vi "Load And Parse Bitfile Test.vi"() -> ()   [LabVIEW 2018]
uses:
  <vilib>/rvi/DataTransferAndStorage/Container/XNode/niFpgaContainer.xnode
  <vilib>/rvi/interface/RandomDataEmulation/nirviRandomDataFpgaReadWriteTemplate.vi
panel:
  out "Fast timeout 3":bool
  out "Fast timeout 2":bool
  in  "Group1.I16":i16
  in  "Group1.I8":i8
  in  "Group1.I64":i64
  in  "Group1.I32":i32
  in  "Group1.U16":u16
  in  "Group1.U8":u8
  in  "Group1.U64":u64
  in  "Group1.U32":u32
  in  "Group1.SGL":sgl
  in  "Group2.Boolean":bool
  out "Group1.I16 out":i16
  out "Group1.I8 out":i8
  out "Group1.I64 out":i64
  out "Group1.I32 out":i32
  out "Group1.U16 out":u16
  out "Group1.U8 out":u8
  out "Group1.U64 out":u64
  out "Group1.U32 out":u32
  out "Group1.SGL out":sgl
  out "Group2.Boolean out":bool
  in  "Group2.FXP24.5":fxp<+/-,24,5>
  in  "Group2.FXP16.5":fxp<+/-,16,5>
  in  "Group2.FXP32.8":fxp<+/-,32,8>
  in  "Group2.FXP64.32":fxp<+/-,64,32>
  out "Group2.FXP24.5 out":fxp<+/-,24,5>
  out "Group2.FXP16.5 out":fxp<+/-,16,5>
  out "Group2.FXP32.8 out":fxp<+/-,32,8>
  out "Group2.FXP64.32 out":fxp<+/-,64,32>
  in  "Group2.FXP16.7":fxp<+/-,16,7>
  out "Group2.FXP16.7 out":fxp<+/-,16,7>
  in  "Group2.FXP20.5":fxp<+/-,20,5>
  out "Group2.FXP20.5 out":fxp<+/-,20,5>
  in  "Group2.FXP27.5":fxp<+/-,27,5>
  out "Group2.FXP27.5 out":fxp<+/-,27,5>
  in  "Group2.FXP32.16":fxp<+/-,32,16>
  out "Group2.FXP32.16 out":fxp<+/-,32,16>
  in  "Group2.FXP16.3":fxp<+,16,3>
  out "Group2.FXP16.3 out":fxp<+,16,3>
  in  "Group2.FXP18.3":fxp<+,18,3>
  out "Group2.FXP18.3 out":fxp<+,18,3>
  in  "FXP18.3":fxp<+,18,3>
  out "FXP18.3 out":fxp<+,18,3>
  in  "FXP16.3":fxp<+,16,3>
  out "FXP16.3 out":fxp<+,16,3>
  in  "FXP32.16":fxp<+/-,32,16>
  out "FXP32.16 out":fxp<+/-,32,16>
  in  "FXP27.5":fxp<+/-,27,5>
  out "FXP27.5 out":fxp<+/-,27,5>
  in  "FXP20.5":fxp<+/-,20,5>
  out "FXP20.5 out":fxp<+/-,20,5>
  in  "FXP16.7":fxp<+/-,16,7>
  out "FXP16.7 out":fxp<+/-,16,7>
  out "FXP64.32 out":fxp<+/-,64,32>
  out "FXP32.8 out":fxp<+/-,32,8>
  out "FXP16.5 out":fxp<+/-,16,5>
  out "FXP24.5 out":fxp<+/-,24,5>
  in  "FXP64.32":fxp<+/-,64,32>
  in  "FXP32.8":fxp<+/-,32,8>
  in  "FXP16.5":fxp<+/-,16,5>
  in  "FXP24.5":fxp<+/-,24,5>
  out "Fast timeout":bool
  out "Med timeout":bool
  out "Slow timeout":bool
  in  "I16":i16
  in  "I8":i8
  in  "I64":i64
  in  "I32":i32
  in  "U16":u16
  in  "U8":u8
  in  "U64":u64
  in  "U32":u32
  in  "SGL":sgl
  in  "Boolean":bool
  out "I16 out":i16
  out "I8 out":i8
  out "I64 out":i64
  out "I32 out":i32
  out "U16 out":u16
  out "U8 out":u8
  out "U64 out":u64
  out "U32 out":u32
  out "SGL out":sgl
  out "Boolean out":bool
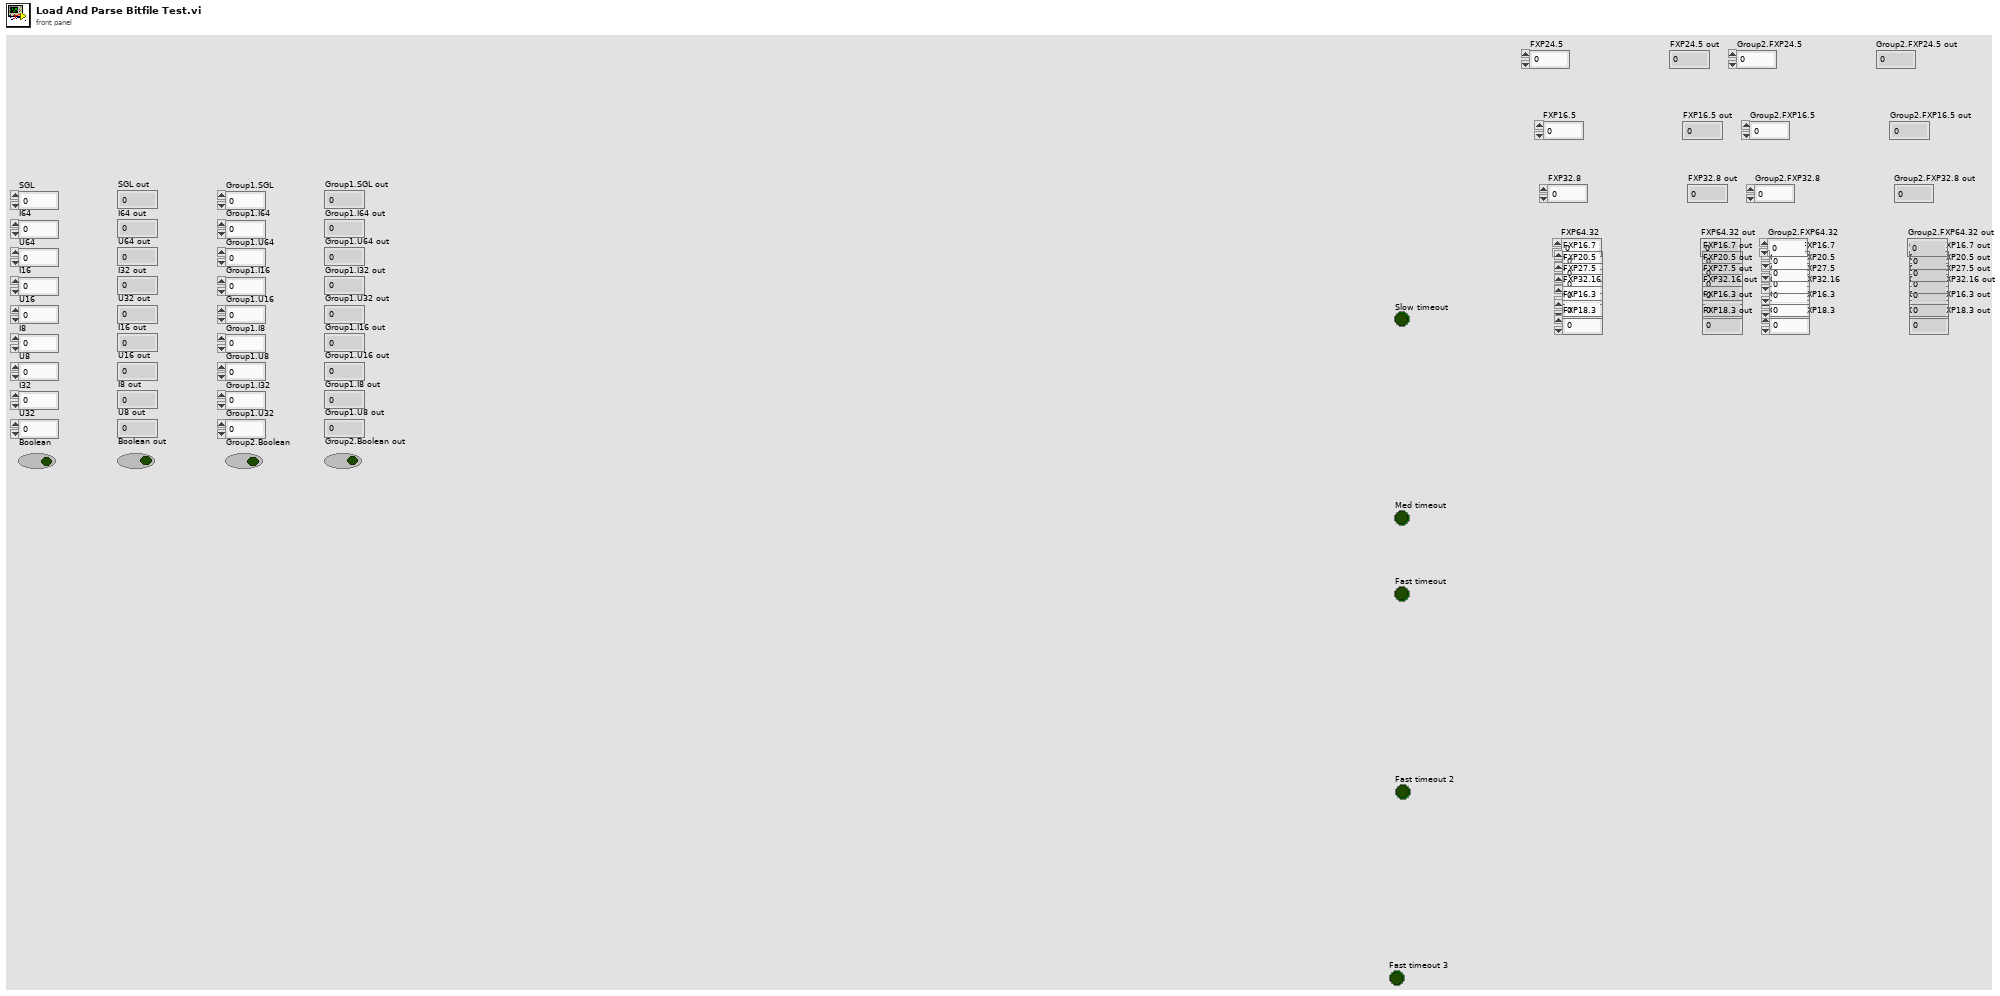
[diagram p1: front panel]
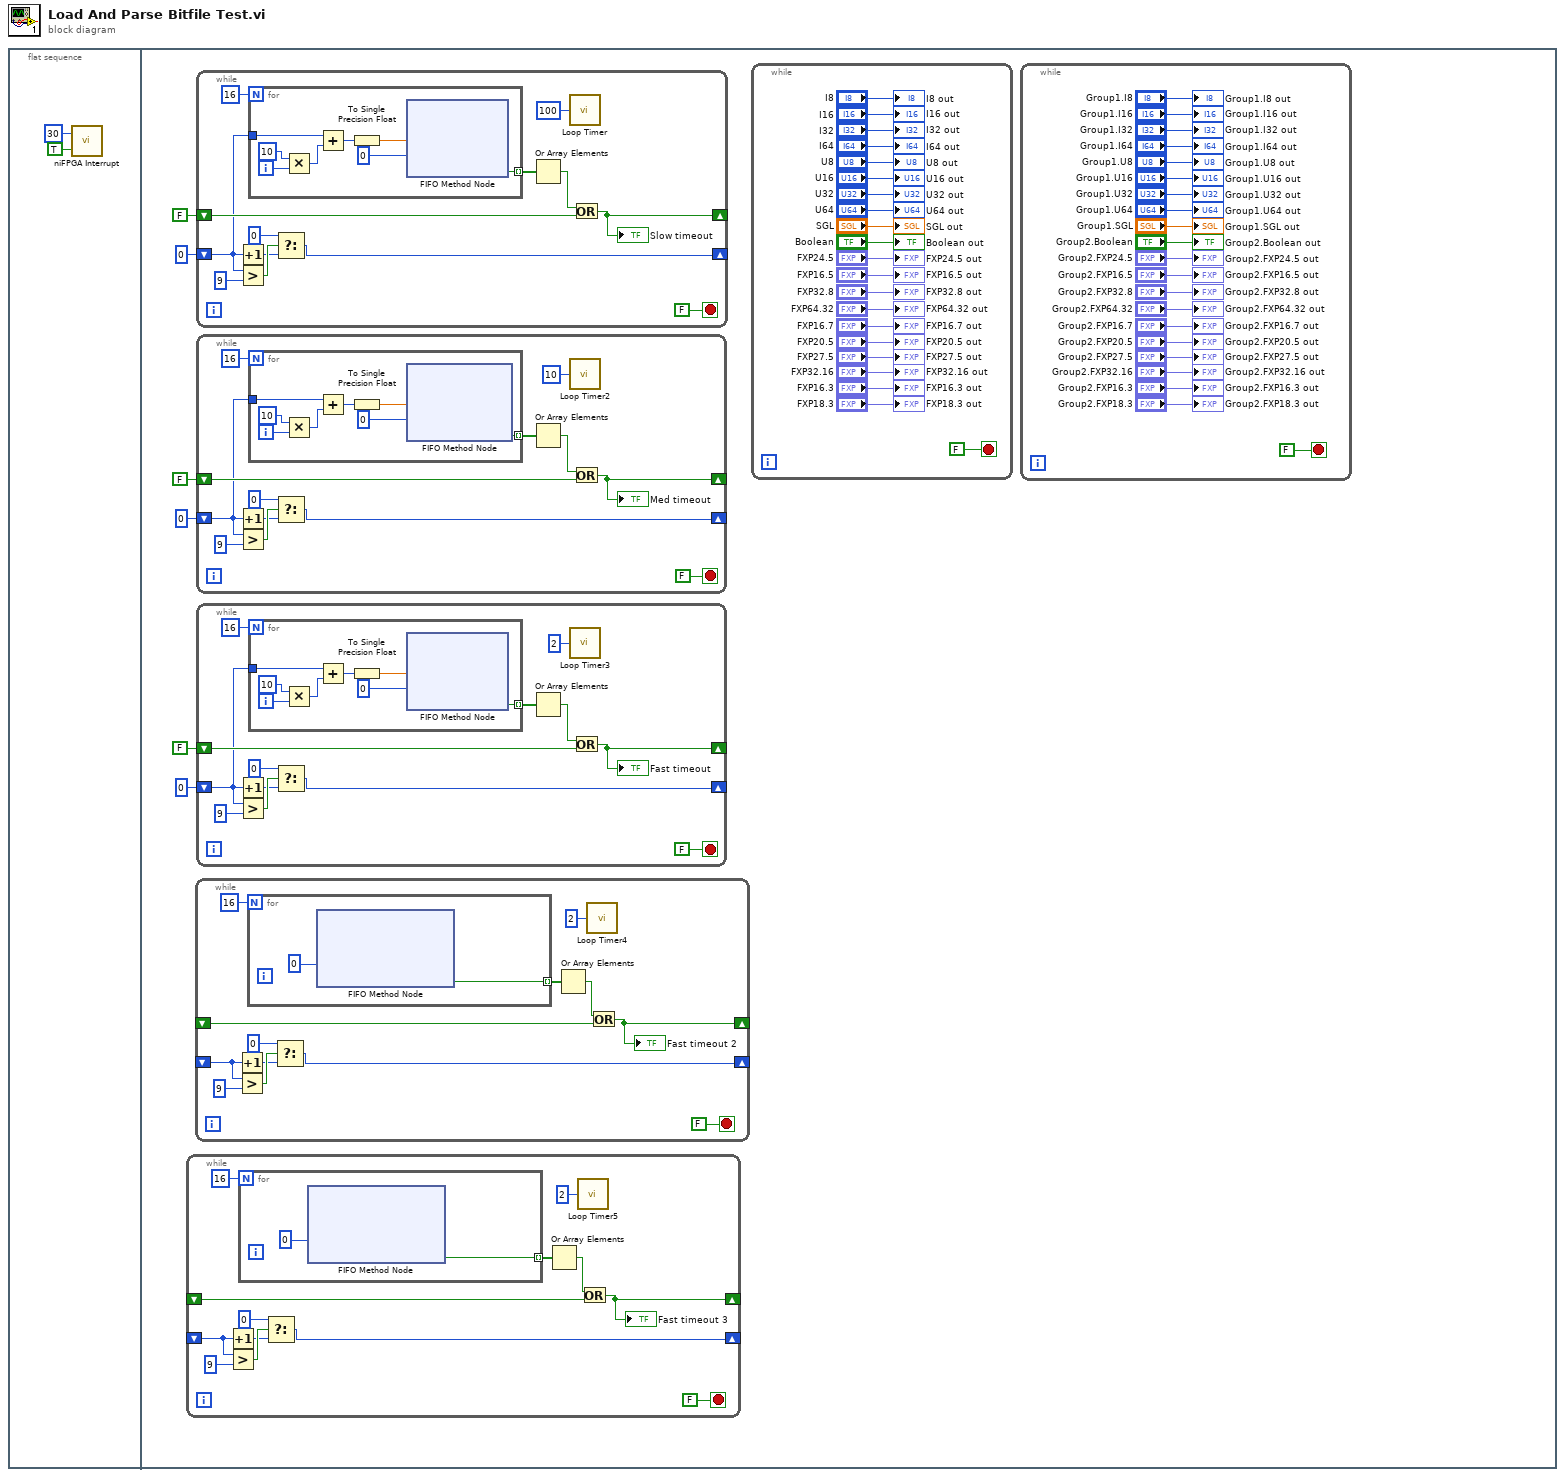
[diagram p0: block diagram]
diagram:
  n1 = flat-sequence {
    frame #0 {
      n2 = call <vilib>:"niFPGA Interrupt.vi"("Wait Until Cleared (F)"=TRUE, "IRQ Number (0)"=u8 30) -> ()  [unwired: 1 in]
    }
    frame #1 {
      n3 = while {
        shift-right: [w16] -> _
        shift-left: _ -> [w10]
        shift-right: [w11] -> _
        shift-left: _ -> [w12]
        stop <- FALSE stop-if-true
        n4 = Increment(x=w10) -> (x+1=w14:i32)
        n5 = Greater?(x=w10, y=9) -> (0:w20:bool)
        n6 = for {
          N: 16 -> [_]
          tunnel: [w22] -> w9 mode=indexing
          n7 = xnode ("FIFO Method Node")("Timeout"=0) -> ("Timed Out?"=w22:bool)  [unwired: 1 in, 2 out]
        }
        n8 = Select(t=0, s=w20, f=w14) -> (s? t:f=w16:i32)
        n9 = Or Array Elements(Boolean array=w9) -> (logical OR=w13:bool)
        n10 = call "Loop Timer5"("Count(uSec)"=u32 2) -> ()  [unwired: 1 out]
        n11 = Or(x=w13, y=w12) -> (x .or. y?=w11:bool)
        "Fast timeout 3" <- w11
      }
      n12 = while {
        shift-right: [w31] -> _
        shift-left: _ -> [w25]
        shift-right: [w26] -> _
        shift-left: _ -> [w27]
        stop <- FALSE stop-if-true
        n13 = Increment(x=w25) -> (x+1=w29:i32)
        n14 = Greater?(x=w25, y=9) -> (0:w35:bool)
        n15 = for {
          N: 16 -> [_]
          tunnel: [w37] -> w24 mode=indexing
          n16 = xnode ("FIFO Method Node")("Timeout"=0) -> ("Timed Out?"=w37:bool)  [unwired: 1 in, 2 out]
        }
        n17 = Select(t=0, s=w35, f=w29) -> (s? t:f=w31:i32)
        n18 = Or Array Elements(Boolean array=w24) -> (logical OR=w28:bool)
        n19 = call "Loop Timer4"("Count(uSec)"=u32 2) -> ()  [unwired: 1 out]
        n20 = Or(x=w28, y=w27) -> (x .or. y?=w26:bool)
        "Fast timeout 2" <- w26
      }
      n21 = while {
        shift-right: [w109] -> _
        shift-left: 0 ("t") -> [w102]
        shift-right: [w103] -> _
        shift-left: FALSE -> [w104]
        stop <- FALSE stop-if-true
        n22 = Increment(x=w102) -> (x+1=w107:i32)
        n23 = Greater?(x=w102, y=9) -> (0:w113:bool)
        n24 = for {
          N: 16 -> [_]
          tunnel: w102 -> [w122]
          tunnel: [w115] -> w106 mode=indexing
          i -> [w121]
          n25 = Multiply(x=10, y=w121) -> (x*y=w119:i32)
          n26 = Add(x=w122, y=w119) -> (x+y=w118:i32)
          n27 = To Single Precision Float(number=w118) -> (single precision float=w117:sgl)
          n28 = xnode ("FIFO Method Node")("Element"=w117, "Timeout"=0) -> ("Timed Out?"=w115:bool)  [unwired: 1 in, 1 out]
        }
        n29 = Select(t=0, s=w113, f=w107) -> (s? t:f=w109:i32)
        n30 = Or Array Elements(Boolean array=w106) -> (logical OR=w105:bool)
        n31 = call "Loop Timer"("Count(uSec)"=u32 100) -> ()  [unwired: 1 out]
        n32 = Or(x=w105, y=w104) -> (x .or. y?=w103:bool)
        "Slow timeout" <- w103
      }
      n33 = while {
        shift-right: [w88] -> _
        shift-left: 0 ("t") -> [w81]
        shift-right: [w82] -> _
        shift-left: FALSE -> [w83]
        stop <- FALSE stop-if-true
        n34 = Increment(x=w81) -> (x+1=w86:i32)
        n35 = Greater?(x=w81, y=9) -> (0:w92:bool)
        n36 = for {
          N: 16 -> [_]
          tunnel: w81 -> [w101]
          tunnel: [w94] -> w85 mode=indexing
          i -> [w100]
          n37 = Multiply(x=10, y=w100) -> (x*y=w98:i32)
          n38 = Add(x=w101, y=w98) -> (x+y=w97:i32)
          n39 = To Single Precision Float(number=w97) -> (single precision float=w96:sgl)
          n40 = xnode ("FIFO Method Node")("Element"=w96, "Timeout"=0) -> ("Timed Out?"=w94:bool)  [unwired: 1 in, 1 out]
        }
        n41 = Select(t=0, s=w92, f=w86) -> (s? t:f=w88:i32)
        n42 = Or Array Elements(Boolean array=w85) -> (logical OR=w84:bool)
        n43 = call "Loop Timer2"("Count(uSec)"=u32 10) -> ()  [unwired: 1 out]
        n44 = Or(x=w84, y=w83) -> (x .or. y?=w82:bool)
        "Med timeout" <- w82
      }
      n45 = while {
        shift-right: [w67] -> _
        shift-left: 0 ("t") -> [w60]
        shift-right: [w61] -> _
        shift-left: FALSE -> [w62]
        stop <- FALSE stop-if-true
        n46 = Increment(x=w60) -> (x+1=w65:i32)
        n47 = Greater?(x=w60, y=9) -> (0:w71:bool)
        n48 = for {
          N: 16 -> [_]
          tunnel: w60 -> [w80]
          tunnel: [w73] -> w64 mode=indexing
          i -> [w79]
          n49 = Multiply(x=10, y=w79) -> (x*y=w77:i32)
          n50 = Add(x=w80, y=w77) -> (x+y=w76:i32)
          n51 = To Single Precision Float(number=w76) -> (single precision float=w75:sgl)
          n52 = xnode ("FIFO Method Node")("Element"=w75, "Timeout"=0) -> ("Timed Out?"=w73:bool)  [unwired: 1 in, 1 out]
        }
        n53 = Select(t=0, s=w71, f=w65) -> (s? t:f=w67:i32)
        n54 = Or Array Elements(Boolean array=w64) -> (logical OR=w63:bool)
        n55 = call "Loop Timer3"("Count(uSec)"=u32 2) -> ()  [unwired: 1 out]
        n56 = Or(x=w63, y=w62) -> (x .or. y?=w61:bool)
        "Fast timeout" <- w61
      }
      n57 = while {
        stop <- FALSE stop-if-true
        "I16 out" <- "I16"
        "I8 out" <- "I8"
        "I64 out" <- "I64"
        "I32 out" <- "I32"
        "U16 out" <- "U16"
        "U8 out" <- "U8"
        "U64 out" <- "U64"
        "U32 out" <- "U32"
        "SGL out" <- "SGL"
        "Boolean out" <- "Boolean"
        "FXP24.5 out" <- "FXP24.5"
        "FXP16.5 out" <- "FXP16.5"
        "FXP32.8 out" <- "FXP32.8"
        "FXP64.32 out" <- "FXP64.32"
        "FXP16.7 out" <- "FXP16.7"
        "FXP20.5 out" <- "FXP20.5"
        "FXP27.5 out" <- "FXP27.5"
        "FXP32.16 out" <- "FXP32.16"
        "FXP16.3 out" <- "FXP16.3"
        "FXP18.3 out" <- "FXP18.3"
      }
      n58 = while {
        stop <- FALSE stop-if-true
        "Group1.I16 out" <- "Group1.I16"
        "Group1.I8 out" <- "Group1.I8"
        "Group1.I64 out" <- "Group1.I64"
        "Group1.I32 out" <- "Group1.I32"
        "Group1.U16 out" <- "Group1.U16"
        "Group1.U8 out" <- "Group1.U8"
        "Group1.U64 out" <- "Group1.U64"
        "Group1.U32 out" <- "Group1.U32"
        "Group1.SGL out" <- "Group1.SGL"
        "Group2.Boolean out" <- "Group2.Boolean"
        "Group2.FXP24.5 out" <- "Group2.FXP24.5"
        "Group2.FXP16.5 out" <- "Group2.FXP16.5"
        "Group2.FXP32.8 out" <- "Group2.FXP32.8"
        "Group2.FXP64.32 out" <- "Group2.FXP64.32"
        "Group2.FXP16.7 out" <- "Group2.FXP16.7"
        "Group2.FXP20.5 out" <- "Group2.FXP20.5"
        "Group2.FXP27.5 out" <- "Group2.FXP27.5"
        "Group2.FXP32.16 out" <- "Group2.FXP32.16"
        "Group2.FXP16.3 out" <- "Group2.FXP16.3"
        "Group2.FXP18.3 out" <- "Group2.FXP18.3"
      }
    }
  }
